vi "FPGA DAC scaling.vi"(7 "DAC update [us]":u32=10 min=1 max=10000 step=1, 8 "Offset 2[Hz]":dbl min=-100000000.0 max=100000000.0 step=10000.0 format="%_3p", 9 "Hz per V2 [Hz]":dbl=500000.0 step=10000.0 format="%_3p", 10 "Offset 1[Hz]":dbl min=-100000000.0 max=100000000.0 step=10000.0 format="%_3p", 11 "Hz per V1 [Hz]":dbl=500000.0 step=10000.0 format="%_3p") -> (0 "offset 2":i16, 1 "scale 2":i16, 2 "offset 1":i16, 3 "scale 1":i16)   [LabVIEW 2014]
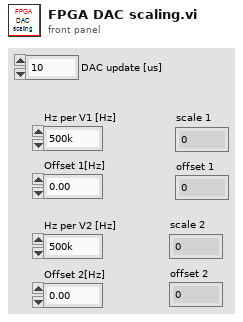
[diagram p1: front panel]
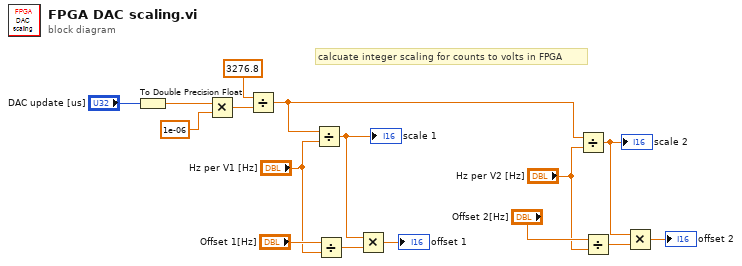
[diagram p0: block diagram]
diagram:
  # "calcuate integer scaling for counts to volts in FPGA"
  n1 = To Double Precision Float(number="DAC update [us]") -> (double precision float=w13:dbl)
  n2 = Multiply(x=w13, y=1e-06) -> (x*y=w10:dbl)
  n3 = Divide(x=3276.8, y=w10) -> (x/y=w5:dbl)
  n4 = Divide(x=w5, y="Hz per V1 [Hz]") -> (x/y=w2:dbl)
  "scale 1" <- w2
  n5 = Divide(x="Offset 1[Hz]", y="Hz per V1 [Hz]") -> (x/y=w14:dbl)
  n6 = Multiply(x=w2, y=w14) -> (x*y=→"offset 1":dbl)
  n7 = Divide(x=w5, y="Hz per V2 [Hz]") -> (x/y=w1:dbl)
  "scale 2" <- w1
  n8 = Divide(x="Offset 2[Hz]", y="Hz per V2 [Hz]") -> (x/y=w7:dbl)
  n9 = Multiply(x=w1, y=w7) -> (x*y=→"offset 2":dbl)
